vi "Call a DLL.vi"() -> ()   [LabVIEW 2025]
uses:
  <resource>/lvanlys.dll
panel:
  out "error out":errorcluster
  in  "error in (no error)":errorcluster
  out "Mean value":dbl
  in  "Input Data":dbl[](array[numeric])=[56.0, 45.0, 67.0, 67.0, 34.0]
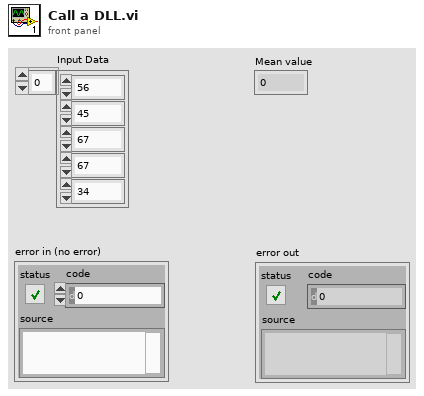
[diagram p1: front panel]
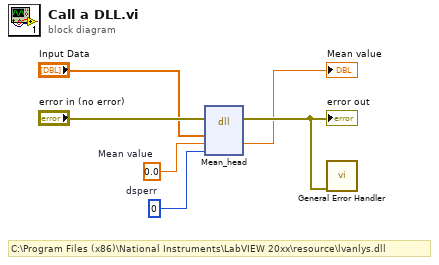
[diagram p0: block diagram]
diagram:
  w1 = 0  # dsperr
  w4 = 0.0  # Mean value
  # "C:\\Program Files (x86)\\National Instruments\\LabVIEW 20xx\\resource\\lvanlys.dll"
  n1 = dll-call lib="D:/Program Files (x86)/National Instruments/LabVIEW 2025/resource/lvanlys.dll" fn="Mean_head"(error in="error in (no error)", "xH"="Input Data", "mean"=w4, "dsperr"=w1) -> (error out=w3:errorcluster, "mean"=→"Mean value":dbl)  [unwired: 5 in, 1 out]
  "error out" <- w3
  n2 = call <vilib>:"General Error Handler.vi"("error in (no error)"=w3) -> ()  [unwired: 10 in, 5 out]
